vi "LKIF2_SetSamplingRate.vi"(8 "error in (no error)":errorcluster, 11 "Sampling Rate":T1) -> (0 "error out":errorcluster)   [LabVIEW 2013, in "Keyence LK-G5000.lvlib"]
uses:
  <instrlib>/Keyence LK-G5000/Keyence LK-G5000.lvlib
  <instrlib>/Keyence LK-G5000/Public/enum/LKIF_SamplingRate.ctl
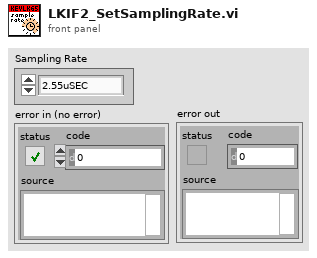
[diagram p1: front panel]
types:
  T1 = typedef "Keyence LK-G5000.lvlib/LKIF_SamplingRate.ctl" = enum16{"2.55uSEC", "5uSEC", "10uSEC", "20uSEC", "50uSEC", "100uSEC", "200uSEC", "500uSEC", "1mSEC"}
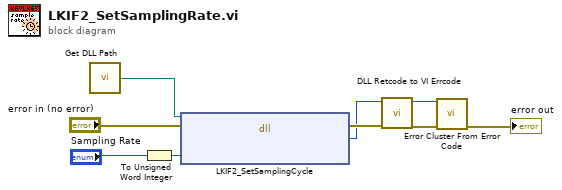
[diagram p0: block diagram]
diagram:
  n1 = call <instrlib>:"Get DLL Path.vi"() -> ("DLL Path"=w6:path)  [unwired: 1 in]
  n2 = To Unsigned Word Integer(number="Sampling Rate") -> (unsigned 16bit integer=w7:u16)
  n3 = dll-call lib="C:/Program Files (x86)/National Instruments/LabVIEW 2013/instr.lib/Keyence LK-G5000/LKIF2.dll" fn="LKIF2_SetSamplingCycle"(path in=w6, error in="error in (no error)", "SamplingCycle"=w7) -> (error out=w5:errorcluster, "RC"=w2:i32)  [unwired: 2 in, 1 out]
  n4 = call <instrlib>:"DLL Retcode to VI Errcode.vi"("error in (no error)"=w5, "DLL Retcode"=w2) -> ("error out"=w8:errorcluster, "VI Errcode"=w9:i32)  [unwired: 8 in]
  n5 = call <vilib>:"Error Cluster From Error Code.vi"("error in (no error)"=w8, "error code (0)"=w9) -> ("error out"=→"error out":errorcluster)  [unwired: 7 in]
